vi "Beregn PWM Servo.vi"(8 "Max (ms puls bredde)":dbl=2.0 format="%#_13g", 9 "Min (ms puls bredde)":dbl=1.0 format="%#_13g", 10 "Duty Cycle":dbl format="%#_13g", 11 "Frekvens":dbl=250.0 format="%#_13g") -> (2 "Output Dutycycle til PWM Servo":dbl)   [LabVIEW 2018]
panel:
  out "Min DC":dbl
  out "Max DC":dbl
  in  "DC fra 0 - ?":dbl=100.0 format="%#_13g"
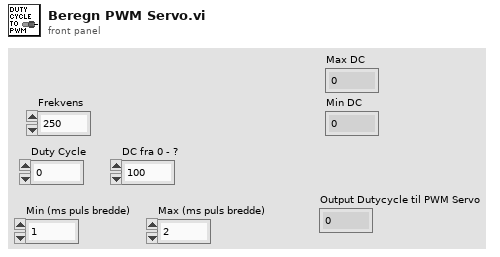
[diagram p1: front panel]
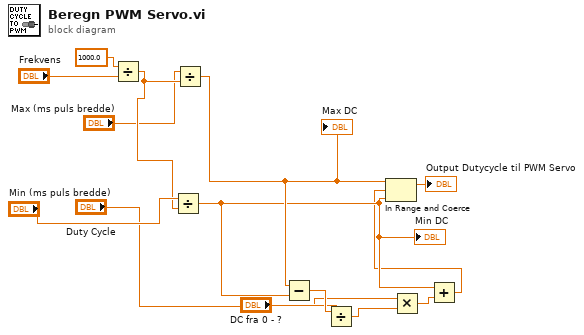
[diagram p0: block diagram]
diagram:
  n1 = Divide(x=1000.0, y="Frekvens") -> (x/y=w11:dbl)
  n2 = Divide(x="Min (ms puls bredde)", y=w11) -> (x/y=w2:dbl)
  "Min DC" <- w2
  n3 = Divide(x="Max (ms puls bredde)", y=w11) -> (x/y=w8:dbl)
  "Max DC" <- w8
  n4 = Subtract(x=w8, y=w2) -> (x-y=w7:dbl)
  n5 = Divide(x=w7, y="DC fra 0 - ?") -> (x/y=w4:dbl)
  n6 = Multiply(x="Duty Cycle", y=w4) -> (x*y=w3:dbl)
  n7 = Add(x=w2, y=w3) -> (x+y=w1:dbl)
  n8 = In Range and Coerce(upper limit=w8, x=w1, lower limit=w2) -> (coerced(x)=→"Output Dutycycle til PWM Servo":dbl)  [unwired: 1 out]
